vi "Eth Status Read Write Enable.vi"(7 "Status Reference":T1, 8 "error in (no error)":errorcluster, 11 "N":i32) -> (0 "error out":errorcluster, 1 "Write Enable":bool)   [LabVIEW 2019, in "Eth Status.lvlib"]
uses:
  Eth Status.lvlib
  Ctl/Status.ctl
  MB_TCP2/MB_TCP_State.ctl
  MB_TCP2/MB_TCP.lvclass
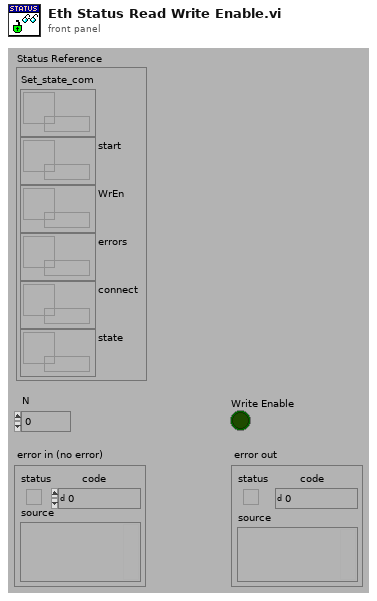
[diagram p1: front panel]
types:
  T1 = typedef "Eth Status.lvlib/Status.ctl" = cluster{"Set_state_com":refnum<data-value>, "start":refnum<data-value>, "WrEn":refnum<data-value>, "errors":refnum<data-value>, "connect":refnum<data-value>, "state":refnum<data-value>}
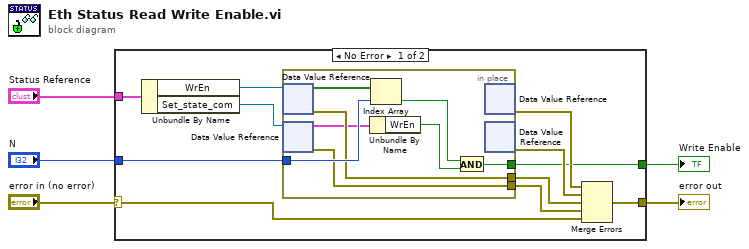
[diagram p0: block diagram]
diagram:
  n1 = case shown="No Error" "error in (no error)" {
    selector: "error in (no error)" -> [w8 w25]
    tunnel: [w7 w25] -> w1
    tunnel: [w6 _] -> w2
    tunnel: "N" -> [w16 _]
    tunnel: "Status Reference" -> [w15 _]
    frame No Error {
      n2 = Unbundle By Name(w15) -> ("WrEn"=w13:refnum<data-value>, "Set_state_com"=w12:refnum<data-value>)
      n3 = in-place {
        in-place-border: w16 -> [w24]
        in-place-border: [w22] -> w10
        in-place-border: [w21] -> w9
        in-place-border: [w17] -> w6
        n4 = in-place-dvr #1(w13) -> (w23:bool[], w22:errorcluster)
        n5 = in-place-dvr #2(w12) -> (w20:cluster{"Start":bool, "WrEn":bool, "Stop":bool}, w21:errorcluster)
        n6 = Unbundle By Name(w20) -> ("WrEn"=w18:bool)
        n7 = Index Array(array=w23, index=w24) -> (element=w19:bool)
        n8 = And(x=w19, y=w18) -> (x .and. y?=w17:bool)
        n9 = in-place-dvr #1() -> (w14:errorcluster)  [unwired: 1 in, 1 out]
        n10 = in-place-dvr #2() -> (w11:errorcluster)  [unwired: 1 in, 1 out]
      }
      n11 = Merge Errors(w14, w11, w10, w9, w8) -> (w7:errorcluster)
    }
    frame Error {
    }
  }
  "error out" <- w1
  "Write Enable" <- w2
